vi "global_variable.vi"() -> ()   [LabVIEW 2018]
panel:
  in  "speed":dbl
  in  "gear":dbl
  in  "brake":dbl
  in  "steer":dbl
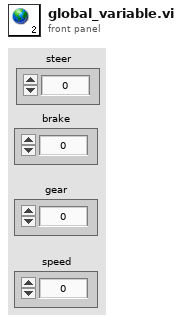
[diagram p1: front panel]
diagram:
